vi "Test 4.vi"() -> ()   [LabVIEW 2016, in "Drona basic.lvlib"]
uses:
  Drona basic.lvlib
  <vilib>/Utility/miscctls.llb/LVPositionTypeDef.ctl
  <vilib>/Utility/miscctls.llb/LVBoundsTypeDef.ctl
panel:
  out "Bounds 2":T1
  out "Position 2":T2
  in  "Cluster":T3 {"Cluster 2"."Cluster 4"."Cluster 3"."Ring" items=["hello", "welcome"]}
  in  "Boolean":bool
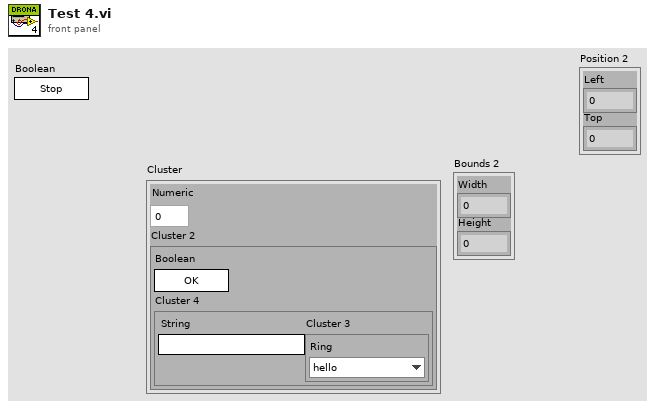
[diagram p1: front panel]
types:
  T1 = typedef "LVBoundsTypeDef.ctl" = cluster{"Width":u32, "Height":u32}
  T2 = typedef "LVPositionTypeDef.ctl" = cluster{"Left":i32, "Top":i32}
  T3 = cluster{"Numeric":dbl, "Cluster 2":cluster{"Boolean":bool, "Cluster 4":cluster{"String":string, "Cluster 3":cluster{"Ring":u16}}}}
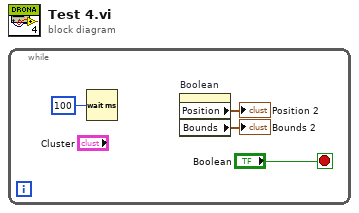
[diagram p0: block diagram]
diagram:
  n1 = while {
    stop <- "Boolean" stop-if-true
    n2 = Wait (ms)(milliseconds to wait=u32 100) -> ()  [unwired: 1 out]
    n3 = property on="Boolean" class="Bool"() -> ("Position"=→"Position 2":T2, "Bounds"=→"Bounds 2":T1)  [unwired: 2 in, 2 out]
  }
